vi "Tektronix INIT.vi"(8 "error in (no error)":errorcluster, 11 "Datos Osciloscopio":T1={"Sesión Visa Osciloscopio"="Tektronix_TDS2012C", "Tipo de Adquisición"=enum."Voltaje Pico Pico", "Canal a Utilizar"=enum."Canal 1", "Parametros de Adquisición"=enum."Una Muestra", "Número Promedio"=0} {"Número Promedio" min=2 max=20}) -> (0 "error out":errorcluster)   [LabVIEW 2017]
doc: "Este vi configura el osciloscopio para el tipo de adquisición (promedio,una muestra, #de muestras, y que la lectura inmediata sea pico a pico o RMS"
uses:
  Type Definitions/datos osciloscopio.ctl
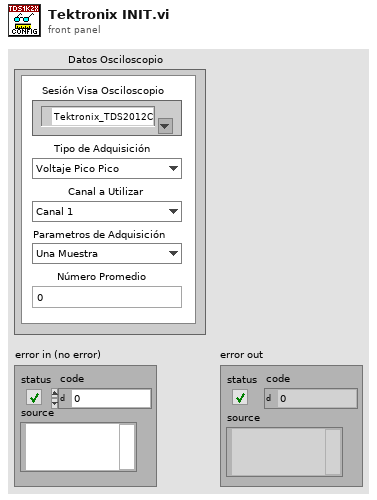
[diagram p1: front panel]
types:
  T1 = typedef "datos osciloscopio.ctl" = cluster{"Sesión Visa Osciloscopio":refnum<visa-resource-name>, "Tipo de Adquisición":enum16{"Voltaje Pico Pico", "Voltaje RMS", "Cursor Tiempo"}, "Canal a Utilizar":enum16{"Canal 1", "Canal 2", "Canal 1 y 2"}, "Parametros de Adquisición":enum16{"Una Muestra", "Promedio"}, "Número Promedio":i32}
  T2 = enum16{"Voltaje Pico Pico", "Voltaje RMS", "Cursor Tiempo"}
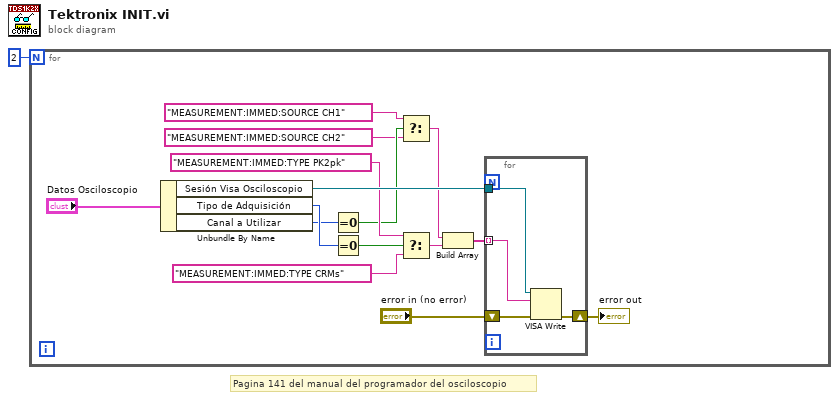
[diagram p0: block diagram]
diagram:
  # "Pagina 141 del manual del programador del osciloscopio"
  n1 = for {
    N: 2 -> [_]
    n2 = Unbundle By Name("Datos Osciloscopio") -> ("Sesión Visa Osciloscopio"=w16:refnum<visa-resource-name>, "Tipo de Adquisición"=w9:T2, "Canal a Utilizar"=w8:enum16{"Canal 1", "Canal 2", "Canal 1 y 2"})
    n3 = Equal To 0?(x=w8) -> (x = 0?=w7:bool)
    n4 = Equal To 0?(x=w9) -> (x = 0?=w12:bool)
    n5 = Select(t="MEASUREMENT:IMMED:SOURCE CH1", s=w7, f="MEASUREMENT:IMMED:SOURCE CH2") -> (s? t:f=w4:string)
    n6 = Select(t="MEASUREMENT:IMMED:TYPE PK2pk", s=w12, f="MEASUREMENT:IMMED:TYPE CRMs") -> (s? t:f=w3:string)
    n7 = Build Array(w4, w3) -> (w2:string[])
    n8 = for {
      tunnel: w16 -> [w20]
      shift-right: [w18] -> w13
      shift-left: "error in (no error)" -> [w19]
      tunnel: w2 -> [w17] mode=indexing
      n9 = VISA Write(VISA resource name=w20, write buffer=w17, error in (no error)=w19) -> (error out=w18:errorcluster)  [unwired: 2 out]
    }
    "error out" <- w13
  }
